vi "Cut.vi"(11 "Accumulator":refnum<class "Accumulator.lvclass">) -> (3 "Accumulator'":refnum<class "Accumulator.lvclass">)   [LabVIEW 2020, in "Accumulator.lvclass"]
uses:
  Accumulator.lvclass
  Accumulator.lvclass/Accumulator.ctl
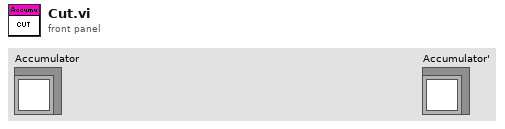
[diagram p1: front panel]
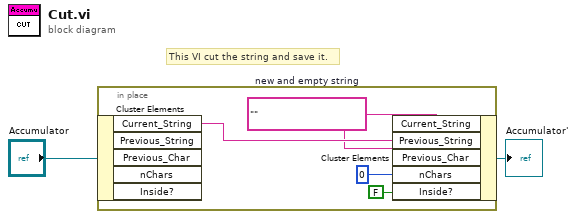
[diagram p0: block diagram]
diagram:
  # "This VI cut the string and save it."
  n1 = in-place {
    w5 = ""  # new and empty string
    n2 = in-place-cluster #1("Accumulator") -> ("Current_String"=w6:string)  [unwired: 4 out]
    n3 = in-place-cluster #1("Current_String"=w5, "Previous_String"=w6, "Previous_Char"=w5, "nChars"=0, "Inside?"=FALSE) -> (→"Accumulator'":refnum<class "Accumulator.lvclass">)
  }
